vi "Handle Error.vi"(8 "error in (no error)":errorcluster, 11 "LeakyViewable in":refnum<class "LeakyViewable.lvclass">) -> (0 "error out":errorcluster, 2 "stop actor?":bool=TRUE, 3 "LeakyViewable out":refnum<class "LeakyViewable.lvclass">)   [LabVIEW 2017, in "ViewableDoubles.lvlib" / "LeakyViewable.lvclass"]
doc: "(<B>Filename</B>: Actor Framework.lvlib:Actor.lvclass:Handle Error.vi)\n\nDefines how the actor handles an error that occurred while processing a message. By default, this method does nothing except stop the actor."
uses:
  LeakyViewable.lvclass
  Leak Location.ctl
  Source/Framework/IViewable/IViewable/IViewable.lvclass
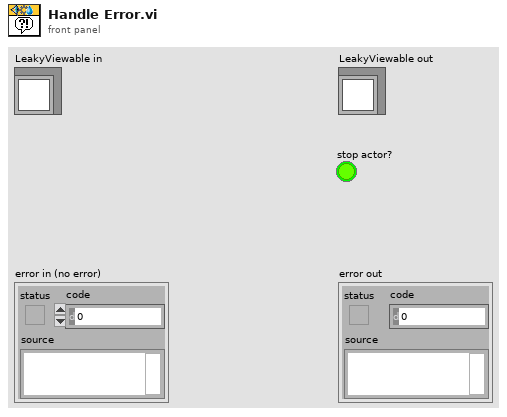
[diagram p1: front panel]
types:
  T1 = typedef "ViewableDoubles.lvlib/LeakyViewable.lvclass/Leak Location.ctl" = enum16{"Pre Launch Init", "Entering Actor Core", "Actor Core", "Exiting Actor Core", "Stop Core", "Handle Error"}
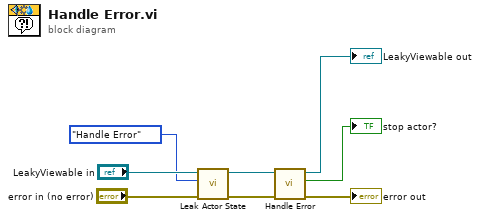
[diagram p0: block diagram]
diagram:
  n1 = call "Leak Actor State.vi"("error in (no error)"="error in (no error)", "Location"=Leak_Location."Handle Error", "ViewableOne in"="LeakyViewable in") -> ("error out"=w4:errorcluster, "ViewableOne out"=w2:refnum<class "LeakyViewable.lvclass">)  [unwired: 7 in]
  n2 = call-parent "Handle Error.vi"("error in (no error)"=w4, "IObserver in"=w2) -> ("error out"=→"error out":errorcluster, "stop actor?"=→"stop actor?":bool, "IObserver out"=→"LeakyViewable out":refnum<class "LeakyViewable.lvclass">)  [unwired: 7 in]
